vi "double_2u16.vi"(11 "Entrada":sgl) -> (0 "Salida 2":u16, 3 "Salida 1":u16)   [LabVIEW 2021]
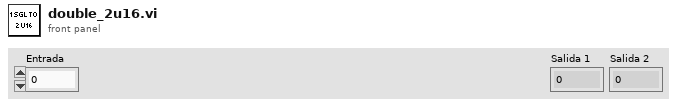
[diagram p1: front panel]
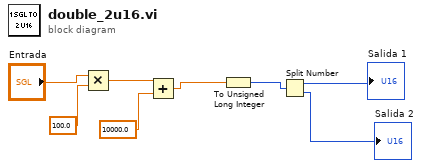
[diagram p0: block diagram]
diagram:
  n1 = Multiply(x="Entrada", y=sgl 100.0) -> (x*y=w3:sgl)
  n2 = Add(x=w3, y=sgl 10000.0) -> (x+y=w2:sgl)
  n3 = To Unsigned Long Integer(number=w2) -> (unsigned 32bit integer=w6:u32)
  n4 = Split Number(x=w6) -> (hi(x)=→"Salida 1":u16, lo(x)=→"Salida 2":u16)
